vi "runscenario.vi"(7 "httpRequestID":u32) -> ()   [LabVIEW 2011]
doc: "This VI is a state machine that can be ran from a Browser."
uses:
  server/database/Users/User Record.ctl
  <vilib>/wsapi/NI_WebServices.lvlib
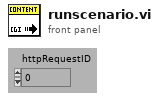
[diagram p1: front panel]
types:
  T1 = typedef "User Record.ctl" = cluster{"ixUser":i32, "sxUsername":string, "sLastName":string, "sFirstName":string, "sEmail":string, "sPassword":string, "tLoginTime":timestamp, "sLoginComputer":string, "fAdministrator":bool, "fRunSequences":bool, "fModifySequences":bool, "fRunScenarios":bool, "fModifyScenarios":bool, "fModifyTemplates":bool, "fModifyUsers":bool, "fModifyStations":bool, "fModifyFields":bool}
  T2 = typedef "Connection Refnum.ctl" = cluster{"Environment Handle":i32, "Connection Handle":i32}
  T3 = typedef "Keyed Array.ctl" = cluster{"keys":string[], "values":string[]}
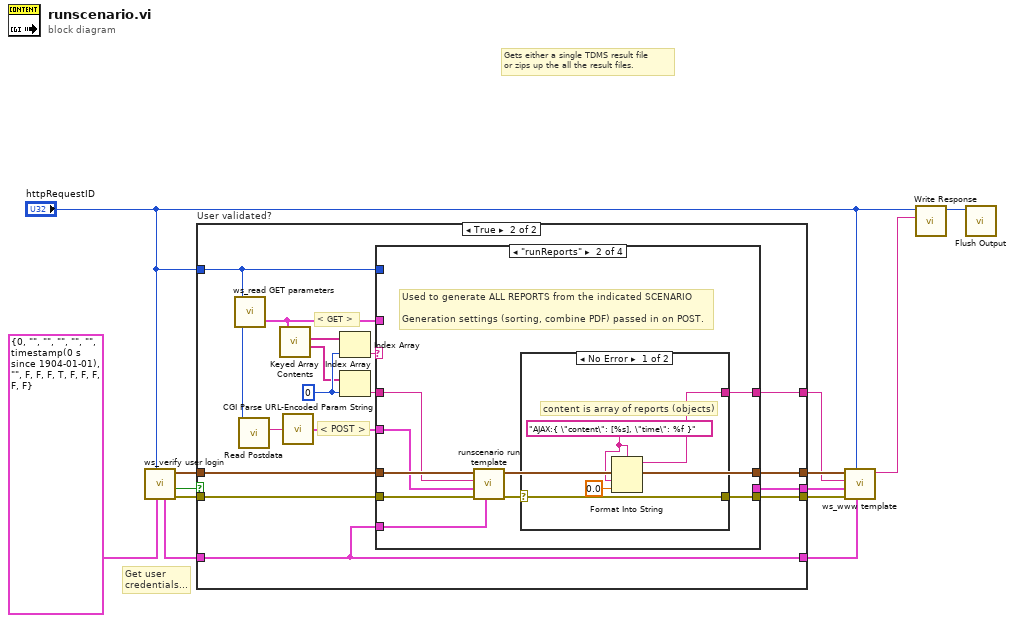
[diagram p0: block diagram]
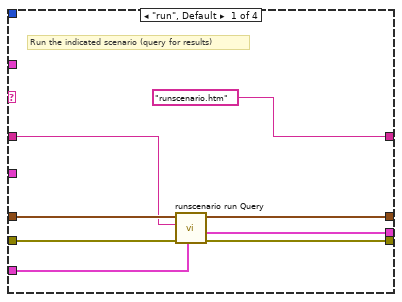
[diagram p3: hidden frame]
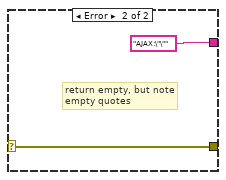
[diagram p4: hidden frame]
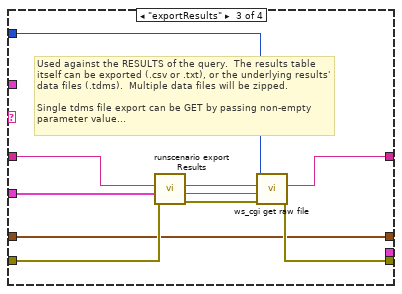
[diagram p5: hidden frame]
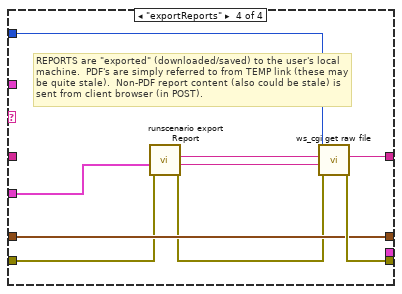
[diagram p6: hidden frame]
diagram:
  # "Gets either a single TDMS result file\nor zips up the all the result files."
  # "Get user \ncredentials..."
  n1 = call "ws_verify user login.vi"("Required Permisions"=T1 {"ixUser"=0, "sxUsername"="", "sLastName"="", "sFirstName"="", "sEmail"="", "sPassword"="", "tLoginTime"=timestamp(0 s since 1904-01-01), "sLoginComputer"="", "fAdministrator"=FALSE, "fRunSequences"=FALSE, "fModifySequences"=FALSE, "fRunScenarios"=TRUE, "fModifyScenarios"=FALSE, "fModifyTemplates"=FALSE, "fModifyUsers"=FALSE, "fModifyStations"=FALSE, "fModifyFields"=FALSE}, "httpRequestID"="httpRequestID") -> ("error out"=w6:errorcluster, "User Verified\nand Spartan\nAuthorized?"=w3:bool, "DB Connection Ref"=w2:T2, "User"=w5:T1)  [unwired: 6 in]
  n2 = case "User validated?" shown="True" w3 {
    tunnel: w5 -> [w15 w23]
    tunnel: w2 -> [w14 w25]
    tunnel: w6 -> [w16 w24]
    tunnel: [w16 w22] -> w12
    tunnel: [w14 w26] -> w13
    tunnel: [_ w20] -> w11
    tunnel: [w15 w23] -> w9
    tunnel: [_ w21] -> w10
    tunnel: "httpRequestID" -> [_ w17]
    frame False {
    }
    frame True {
      w29 = 0 ("index")
      # "< GET >"
      # "< POST >"
      n3 = call "ws_read GET parameters.vi"("httpRequestID"=w17) -> ("GET query params"=w19:T3)  [unwired: 2 in]
      n4 = call <vilib>:"Read Postdata.vi"("httpRequestID"=w17) -> ("postdata"=w18:string)  [unwired: 8 in, 2 out]
      n5 = call <vilib>:"Keyed Array Contents.vi"("array in"=w19) -> ("values"=w28:string[], "keys"=w30:string[])  [unwired: 4 in, 1 out]
      n6 = call <vilib>:"CGI Parse URL-Encoded Param String.vi"("url-encoded param string"=w18) -> ("params"=w32:T3)
      n7 = Index Array(array=w30, index=w29) -> (element=w31:string)
      n8 = Index Array(array=w28, index=w29) -> (element=w27:string)
      n9 = case shown="\"runReports\"" w31 {
        tunnel: [w33 w42 w65 w74] -> w22
        tunnel: w24 -> [w38 w49 w63 w71]
        tunnel: w23 -> [w34 w48 _ _]
        tunnel: ["runscenario.htm" w44 w64 w73] -> w20
        tunnel: [w35 _ _ _] -> w21
        tunnel: w32 -> [_ w41 w60 w70]
        tunnel: w19 -> [_ _ _ _]
        tunnel: w25 -> [w39 w46 w57 w72]
        tunnel: [w37 w47 w57 w72] -> w26
        tunnel: w27 -> [w36 w45 w61 _]
        tunnel: w17 -> [_ _ w56 w66]
        frame "run", Default {
          # "Run the indicated scenario (query for results)"
          n10 = call "runscenario run Query.vi"("User Information"=w34, "error in (no error)"=w38, "sxScenarioId (\"\")"=w36, "Connection Refnum In"=w39) -> ("error out"=w33:errorcluster, "template keys"=w35:T3, "Connection Refnum Out"=w37:T2)  [unwired: 1 in, 4 out]
        }
        frame "runReports" {
          # "Used to generate ALL REPORTS from the indicated SCENARIO\n\nGeneration settings (sorting, combine PDF) passed in on POST."
          n11 = call "runscenario run template.vi"("User Information"=w48, "error in (no error)"=w49, "POST (empty)"=w41, "sxScenarioId (\"\")"=w45, "Connection Refnum"=w46) -> ("error out"=w43:errorcluster, "dup Connection Refnum"=w47:T2)  [unwired: 1 in, 4 out]
          n12 = case shown="No Error" w43 {
            selector: w43 -> [w52 w55]
            tunnel: [w53 "AJAX:\"\""] -> w44
            tunnel: [w52 w55] -> w42
            frame No Error {
              w51 = "AJAX:{ \"content\": [%s], \"time\": %f }" ("Template (\"\")")
              # "content is array of reports (objects)"
              n13 = Format Into String(format string=w51, w51, 0.0 ("input 2")) -> (resulting string=w53:string)  [unwired: 2 in, 1 out]
            }
            frame Error {
              # "return empty, but note\nempty quotes"
            }
          }
        }
        frame "exportResults" {
          # "Used against the RESULTS of the query.  The results table\nitself can be exported (.csv or .txt), or the underlying results'\ndata files (.tdms).  Multiple data files will be zipped.\n\nSingle tdms file export can be GET by passing non-empty\nparameter value..."
          n14 = call "runscenario export Results.vi"("error in (no error)"=w63, "POST (empty)"=w60, "GET Parameter (\"\")"=w61) -> ("error out"=w62:errorcluster, "Filename"=w58:string, "Content"=w59:string)  [unwired: 2 in, 4 out]
          n15 = call "ws_cgi get raw file.vi"("error in (no error)"=w62, "Filename (\"\")"=w58, "Content (\"\")"=w59, "httpRequestID"=w56) -> ("error out"=w65:errorcluster, "Packed Content"=w64:string)  [unwired: 6 in]
        }
        frame "exportReports" {
          # "REPORTS are \"exported\" (downloaded/saved) to the user's local\nmachine.  PDF's are simply referred to from TEMP link (these may\nbe quite stale).  Non-PDF report content (also could be stale) is\nsent from client browser (in POST)."
          n16 = call "runscenario export Report.vi"("error in (no error)"=w71, "POST (empty)"=w70) -> ("error out"=w67:errorcluster, "Export Filename"=w68:string, "Export Content"=w69:string)  [unwired: 2 in, 5 out]
          n17 = call "ws_cgi get raw file.vi"("error in (no error)"=w67, "Filename (\"\")"=w68, "Content (\"\")"=w69, "httpRequestID"=w66) -> ("error out"=w74:errorcluster, "Packed Content"=w73:string)  [unwired: 6 in]
        }
      }
    }
  }
  n18 = call "ws_www template.vi"("User"=w9, "httpRequestID"="httpRequestID", "error in (no error)"=w12, "Template Keys (empty)"=w10, "Template (\"\")"=w11, "DB Connection Ref"=w13) -> ("HTTP Template Content"=w8:string)  [unwired: 5 in]
  n19 = call <vilib>:"Write Response.vi"("response string"=w8, "httpRequestID"="httpRequestID") -> ("httpRequestID out"=w7:u32)  [unwired: 8 in, 1 out]
  n20 = call <vilib>:"Flush Output.vi"("httpRequestID"=w7) -> ()  [unwired: 9 in, 2 out]
